vi "Set Output.vi"(8 "error in (no error)":errorcluster, 10 "Output value":refnum<class "Output Value.lvclass">, 11 "Spectrum Recorder in":refnum<class "Spectrum Recorder too.lvclass">) -> (0 "error out":errorcluster, 3 "Spectrum Recorder out":refnum<class "Spectrum Recorder too.lvclass">)   [LabVIEW 2019, in "Spectrum Recorder too.lvclass"]
uses:
  Spectrum Recorder too.lvclass
  NHMFL_Core/Libraries/Utilities/Output Value/Output Value.lvclass
  Instrument Actor/Instrument Actor.lvclass
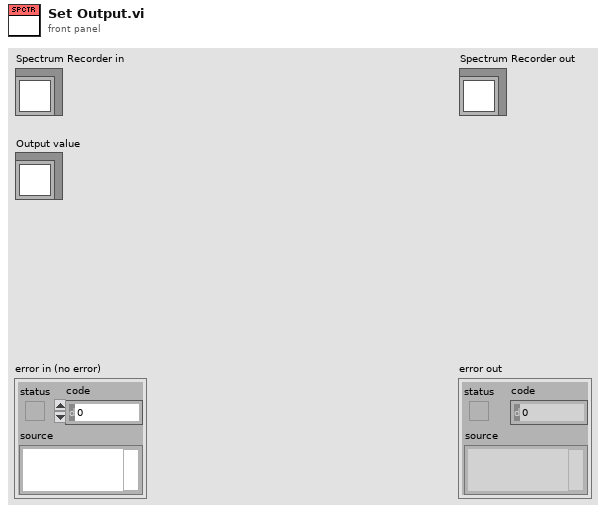
[diagram p1: front panel]
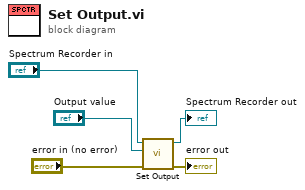
[diagram p0: block diagram]
diagram:
  n1 = call-parent "Set Output.vi"("error in (no error)"="error in (no error)", "Output value"="Output value", "Instrument Actor in"="Spectrum Recorder in") -> ("error out"=→"error out":errorcluster, "Instrument Actor out"=→"Spectrum Recorder out":refnum<class "Spectrum Recorder too.lvclass">)  [unwired: 7 in]
